vi "Configure Alarm IO.vi"(0 "VISA resource name":refnum<visa-resource-name>, 1 "Alarm Type (1 : High limit alarm)":i32(ring)=1 items=["High Limit Alarm (H)"=1, "Low Limit Alarm (L)"=2, "Difference High Limit Alarm (h)"=3, "Difference Low Limit Alarm (l)"=4, "High Limit on Rate-of-change Alarm (R)"=5, "Low Limit on Rate-of-change Alarm (r)"=6, "Delay High Limit Alarm (T)"=7, "Delay Low Limit Alarm (t)"=8], 2 "Alarm Value (0)":i32 min=-99999999 max=99999999 step=1 format="%#_8g", 3 "Enable Detect (False)":bool, 5 "Channel (0001)":string="0001", 7 "Enable Alarm (False)":bool, 9 "Alarm Number (1)":i32=1 min=1 max=4 step=1, 11 "error in (no error)":errorcluster, 12 "Output Type (0: Off)":u16(ring) items=["Off", "DO", "Internal Switch"], 13 "DO/Switch Number (0001)":string="0001", 14 "Alarm Value For Log Calc (0)":dbl format="%.2e") -> (4 "VISA resource name out":refnum<visa-resource-name>, 6 "Channel":string, 8 "Alarm Number":i32, 15 "error out":errorcluster)   [LabVIEW 2020, in "Yokogawa GX Series.lvlib"]
doc: "Sets the alarm for AI and DI channels.\n\nCommand: SAlarmIO"
uses:
  <instrlib>/Yokogawa GX Series/Yokogawa GX Series.lvlib
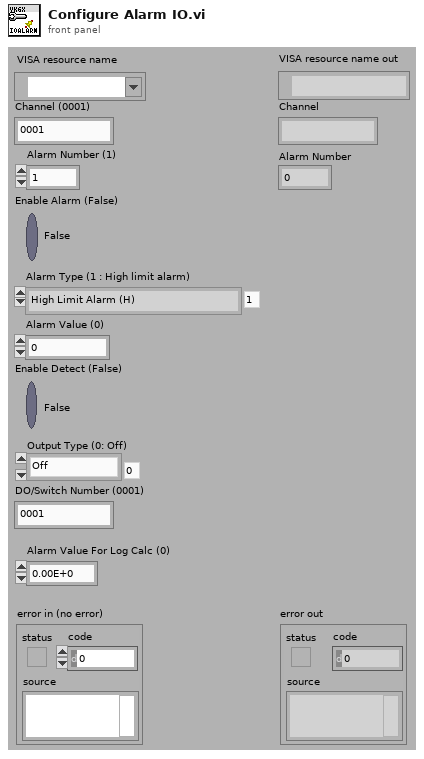
[diagram p1: front panel]
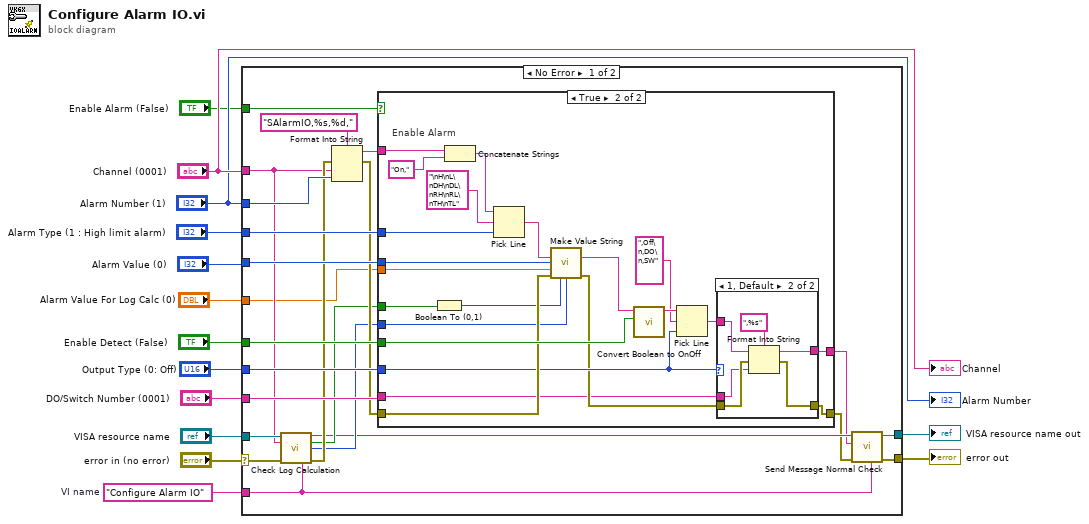
[diagram p0: block diagram]
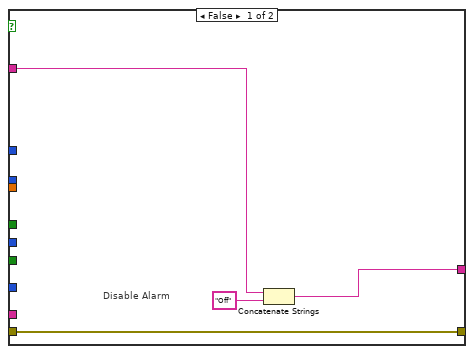
[diagram p2: hidden frame]
diagram:
  w11 = "Configure Alarm IO"  # VI name
  n1 = case shown="No Error" "error in (no error)" {
    selector: "error in (no error)" -> [w27 w72]
    tunnel: "Alarm Type (1 : High limit alarm)" -> [w35 _]
    tunnel: "Alarm Value (0)" -> [w34 _]
    tunnel: "VISA resource name" -> [w28 w73]
    tunnel: w11 -> [w15 _]
    tunnel: [w17 w73] -> w10
    tunnel: [w16 w72] -> w9
    tunnel: "Enable Detect (False)" -> [w33 _]
    tunnel: "DO/Switch Number (0001)" -> [w32 _]
    tunnel: "Channel (0001)" -> [w24 _]
    tunnel: "Output Type (0: Off)" -> [w31 _]
    tunnel: "Alarm Number (1)" -> [w30 _]
    tunnel: "Enable Alarm (False)" -> [w29 _]
    tunnel: "Alarm Value For Log Calc (0)" -> [w21 _]
    frame No Error {
      n2 = call <instrlib>:"Check Log Calculation.vi"("VISA resource name"=w28, "Channel (0001)"=w24, "error in (no error)"=w27, "Source (\"\")"=w15) -> ("VISA resource name out"=w20:refnum<visa-resource-name>, "Result"=w23:bool, "Float Position"=w22:i32, "error out"=w26:errorcluster)  [unwired: 8 in]
      n3 = Format Into String(format string="SAlarmIO,%s,%d,", error in=w26, w24, w30) -> (resulting string=w36:string, error out=w25:errorcluster)  [unwired: 1 in]
      n4 = case shown="True" w29 {
        tunnel: w36 -> [w40 w61]
        tunnel: w35 -> [_ w62]
        tunnel: w34 -> [_ w54]
        tunnel: w25 -> [w39 w52]
        tunnel: w33 -> [_ w58]
        tunnel: w32 -> [_ w42]
        tunnel: w31 -> [_ w47]
        tunnel: w23 -> [_ w51]
        tunnel: w22 -> [_ w49]
        tunnel: w21 -> [_ w53]
        tunnel: [w39 w45] -> w19
        tunnel: [w38 w43] -> w18
        frame False {
          # "Disable Alarm"
          n5 = Concatenate Strings(w40, "Off") -> (w38:string)
        }
        frame True {
          # "Enable Alarm"
          n6 = Boolean To (0,1)(Boolean=w51) -> (0, 1=w50:i16)
          n7 = Concatenate Strings(w61, "On,") -> (w59:string)
          n8 = Pick Line(string ("")=w59, multi-line string="\nH\nL\nDH\nDL\nRH\nRL\nTH\nTL", line index=w62) -> (output string=w55:string)
          n9 = call <instrlib>:"Make Value String.vi"("Initial String (\"\")"=w55, "Int Value (0)"=w54, "Float Value (0)"=w53, "Error In"=w52, "Kind Of Value (0: Int)"=w50, "Float Decimal Position (1)"=w49) -> ("Resulting String"=w48:string, "Error Out"=w46:errorcluster)  [unwired: 8 in]
          n10 = call <instrlib>:"Convert Boolean to OnOff.vi"("On/Off"=w58, "Initial String (\"\")"=w48) -> ("Resulting String"=w57:string)  [unwired: 9 in]
          n11 = Pick Line(string ("")=w57, multi-line string=",Off\n,DO\n,SW", line index=w47) -> (output string=w44:string)
          n12 = case shown="1, Default" w47 {
            tunnel: w46 -> [w65 w71]
            tunnel: [w65 w66] -> w45
            tunnel: w44 -> [w64 w70]
            tunnel: [w64 w67] -> w43
            tunnel: w42 -> [_ w68]
            frame 0 {
            }
            frame 1, Default {
              n13 = Format Into String(format string=",%s", initial string=w70, error in=w71, w68) -> (resulting string=w67:string, error out=w66:errorcluster)
            }
          }
        }
      }
      n14 = call <instrlib>:"Send Message Normal Check.vi"("Source (\"\")"=w15, "error in (no error)"=w19, "Send Message (\"\")"=w18, "VISA resource name"=w20) -> ("error out"=w16:errorcluster, "VISA resource name out"=w17:refnum<visa-resource-name>)  [unwired: 2 in, 4 out]
    }
    frame Error {
    }
  }
  "error out" <- w9
  "VISA resource name out" <- w10
  "Alarm Number" <- "Alarm Number (1)"
  "Channel" <- "Channel (0001)"
